vi "PrepareInlineData.vi"(8 "error in (no error)":errorcluster, 10 "Inline Data":string, 11 "VI Refnum":refnum<vi>) -> (0 "error out":errorcluster, 1 "Control Data":T1[](array[typedef]), 2 "Data Name":string)   [LabVIEW 2017, in "LVUnitTestBuilder.lvclass"]
uses:
  LVUnitTestBuilder.lvclass
  65fd24c9-a785-4dc1-8b48-2da962c35a9e.vi
  d55797c9-58c8-4118-a156-a05c24b3ba98.vi
  ControlData.ctl
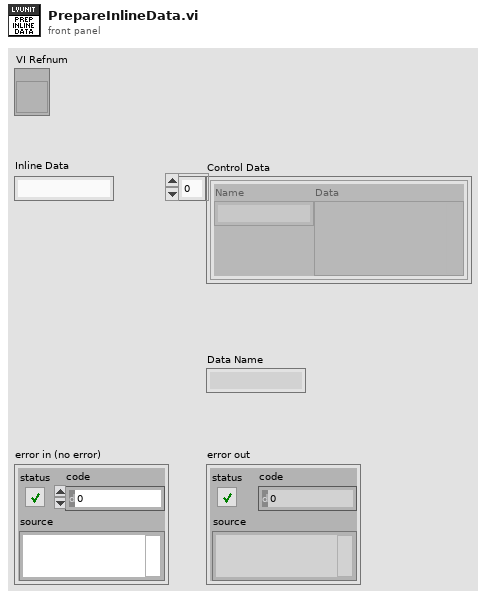
[diagram p1: front panel]
types:
  T1 = typedef "ControlData.ctl" = cluster{"Name":string, "Data":variant}
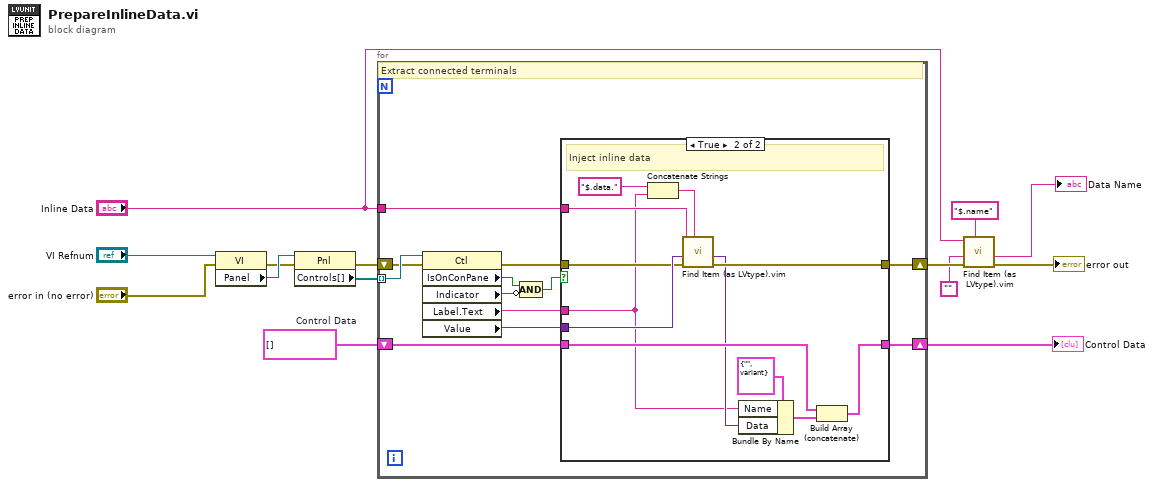
[diagram p0: block diagram]
diagram:
  w1 = T1[] []  # Control Data
  n1 = property class="VI"(reference="VI Refnum", error in="error in (no error)") -> (error out=w13:errorcluster, "Panel"=w14:refnum<vi>)  [unwired: 1 out]
  n2 = property class="Pnl"(reference=w14, error in=w13) -> (error out=w11:errorcluster, "Controls[]"=w12:refnum<vi>[])  [unwired: 1 out]
  n3 = for {
    tunnel: w12 -> [w26] mode=indexing
    shift-right: [w18] -> w9
    shift-left: w11 -> [w25]
    shift-right: [w24] -> w3
    shift-left: w1 -> [w23]
    tunnel: "Inline Data" -> [w19]
    # "Extract connected terminals"
    n4 = property class="Ctl"(reference=w26, error in=w25) -> (error out=w20:errorcluster, "IsOnConPane"=w16:bool, "Indicator"=w17:bool, "Label.Text"=w22:string, "Value"=w21:variant)  [unwired: 1 out]
    n5 = Compound Arithmetic op=AND(w16, invert w17) -> (w15:bool)
    n6 = case shown="True" w15 {
      tunnel: [w28 w40] -> w24
      tunnel: w23 -> [w28 w33]
      tunnel: w22 -> [_ w29]
      tunnel: w21 -> [_ w37]
      tunnel: w20 -> [w27 w36]
      tunnel: [w27 w35] -> w18
      tunnel: w19 -> [_ w34]
      frame False {
      }
      frame True {
        # "Inject inline data"
        n7 = Concatenate Strings("$.data." ("string"), w29) -> (w39:string)
        n8 = call "Find Item (as LVtype).vim"("$Path or Item Name"=w39, "error in (no error)"=w36, "Data Type and Default Value"=w37, "JSON"=w34) -> ("error out"=w35:errorcluster, "Data"=w30:variant)  [unwired: 4 in, 2 out]
        n9 = Bundle By Name(cluster=T1 {"Name"="", "Data"=variant} ("Control Data"), "Name"=w29, "Data"=w30) -> (w31:T1)
        n10 = Build Array (concatenate)(w33, w31) -> (w40:T1[])
      }
    }
  }
  "Control Data" <- w3
  n11 = call "Find Item (as LVtype).vim"("$Path or Item Name"="$.name", "error in (no error)"=w9, "Data Type and Default Value"="", "JSON"="Inline Data") -> ("error out"=→"error out":errorcluster, "Data"=→"Data Name":string)  [unwired: 4 in, 2 out]
